vi "Math_FXPtoI16.vi"(11 "FXP":fxp<+/-,32,16> format="%#_32g") -> (3 "I16":i16)   [LabVIEW 2020]
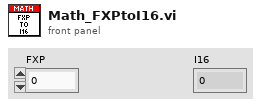
[diagram p1: front panel]
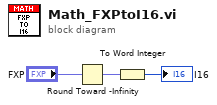
[diagram p0: block diagram]
diagram:
  n1 = Round Toward -Infinity(1:"FXP") -> (0:w3:fxp<+/-,16,16>)
  n2 = To Word Integer(number=w3) -> (16bit integer=→"I16":i16)
